vi "배열.vi"() -> ()   [LabVIEW 2020]
panel:
  out "출력 배열 2":dbl[](array[numeric])
  in  "인덱스 3":dbl
  in  "배열 5":dbl[](array[numeric])
  out "출력 배열":dbl[](array[numeric])
  in  "인덱스 2":dbl
  in  "배열 4":dbl[](array[numeric])
  in  "배열 3":dbl[](array[numeric])
  out "정렬된 배열":dbl[](array[numeric])
  in  "배열 2":dbl[](array[numeric])
  out "원소":dbl
  in  "인덱스":dbl
  in  "배열":dbl[](array[numeric])
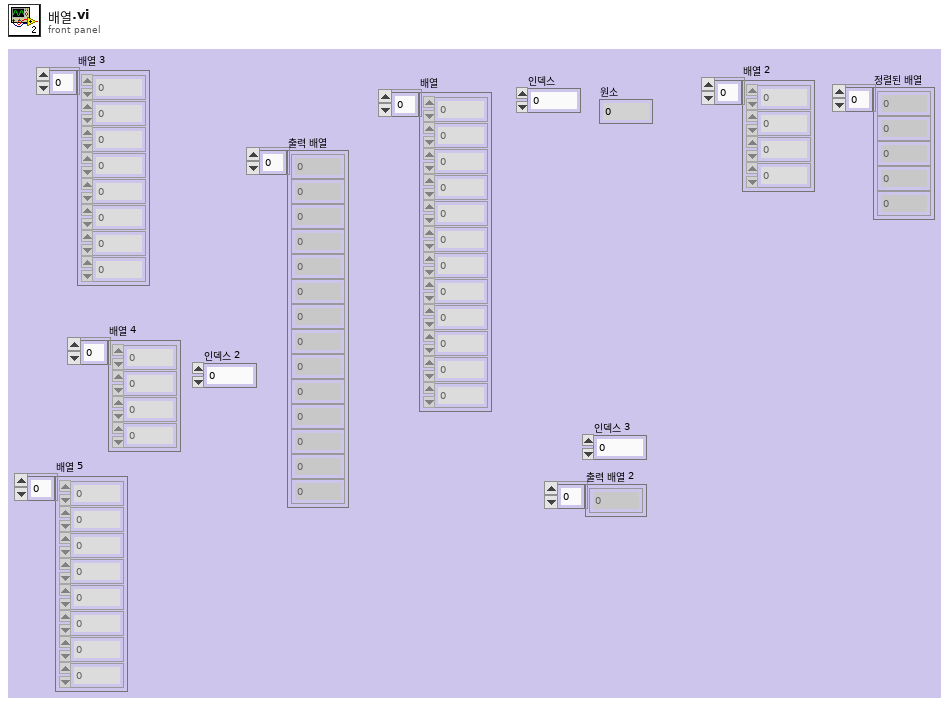
[diagram p1: front panel]
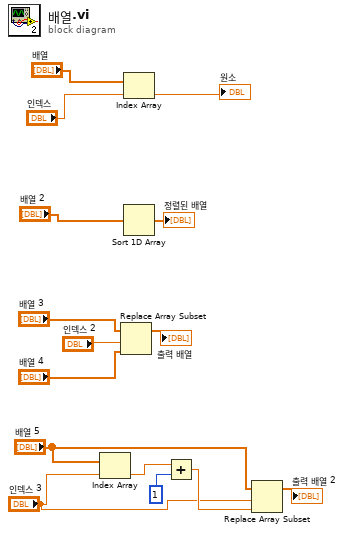
[diagram p0: block diagram]
diagram:
  n1 = Index Array(array="배열 5", index="인덱스 3") -> (element=w5:dbl)
  n2 = Replace Array Subset(array="배열 3", new element="배열 4", index="인덱스 2") -> (→"출력 배열":dbl[])
  n3 = Index Array(array="배열", index="인덱스") -> (element=→"원소":dbl)
  n4 = Sort 1D Array(array="배열 2") -> (sorted array=→"정렬된 배열":dbl[])
  n5 = Add(x=w5, y=1) -> (x+y=w4:dbl)
  n6 = Replace Array Subset(array="배열 5", new element=w4, index="인덱스 3") -> (→"출력 배열 2":dbl[])
